vi "RSNRPZ VXIPnp Error Converter.vi"(2 "error in (no error)":errorcluster {"code" format="%.0x"}, 3 "name of VI":string, 4 "VXIPnp error code":i32, 5 "VISA session":i32) -> (0 "error out":errorcluster {"code" format="%.0x"}, 1 "dup VISA session":i32)   [LabVIEW 2014]
doc: "This VI converts error codes from VXIPnp instrument driver to standard LabVIEW error codes. If an error is detected the VI builds the appropriate error cluster that is readable by one of the error handlers supplied with LabVIEW."
uses:
  rsnrpz_32.dll
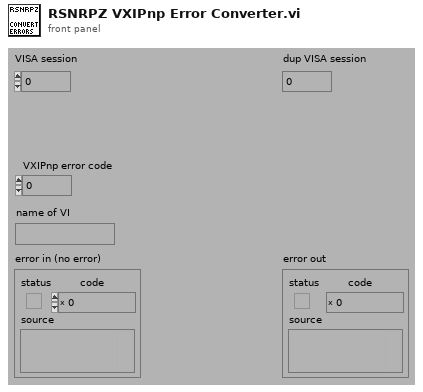
[diagram p1: front panel]
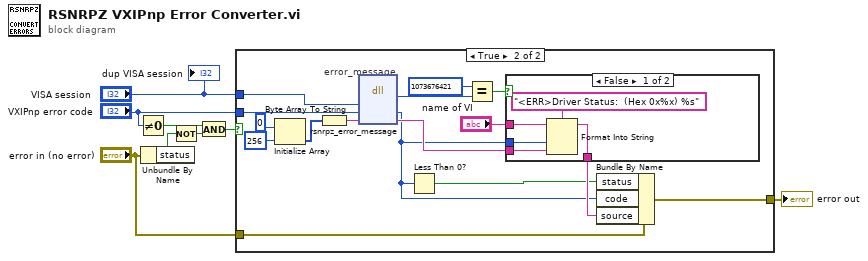
[diagram p0: block diagram]
diagram:
  n1 = Not Equal To 0?(x="VXIPnp error code") -> (x != 0?=w5:bool)
  n2 = Unbundle By Name("error in (no error)") -> ("status"=w4:bool)
  n3 = Not(x=w4) -> (.not. x?=w1:bool)
  n4 = And(x=w5, y=w1) -> (x .and. y?=w3:bool)
  n5 = case shown="True" w3 {
    tunnel: "VXIPnp error code" -> [_ w25]
    tunnel: [w9 w24] -> w8
    tunnel: "error in (no error)" -> [w9 w23]
    tunnel: "VISA session" -> [_ w18]
    frame False {
    }
    frame True {
      # "error_message"
      n6 = Initialize Array(u8 0, 256) -> (w21:u8[])
      n7 = Byte Array To String(unsigned byte array=w21) -> (string=w19:string)
      n8 = dll-call lib="rsnrpz_32.dll" fn="rsnrpz_error_message"("instrumentHandle"=w18, "statusCode"=w25, "message"=w19) -> (w16:i32, "statusCode"=w10:i32, "message"=w14:string)  [unwired: 4 in, 2 out]
      n9 = Less Than 0?(x=w10) -> (x < 0?=w11:bool)
      n10 = Equal?(x=1073676421 ("y"), y=w16) -> (x = y?=w15:bool)
      n11 = case shown="False" w15 {
        tunnel: w14 -> [w28 _]
        tunnel: "name of VI" -> [w30 w31]
        tunnel: w10 -> [w29 _]
        tunnel: [w27 w31] -> w12
        frame False {
          n12 = Format Into String(format string="<ERR>Driver Status:  (Hex 0x%x) %s", initial string=w30, w29, w28) -> (resulting string=w27:string)  [unwired: 1 in, 1 out]
        }
        frame True {
        }
      }
      n13 = Bundle By Name(cluster=w23, "status"=w11, "code"=w10, "source"=w12) -> (w24:errorcluster)
    }
  }
  "error out" <- w8
  "dup VISA session" <- "VISA session"
